vi "WAV_Binarize.vi"(10 "Data in":sgl[][](graph), 11 "format":T1) -> (2 "file string":string)   [LabVIEW 2022 SP3]
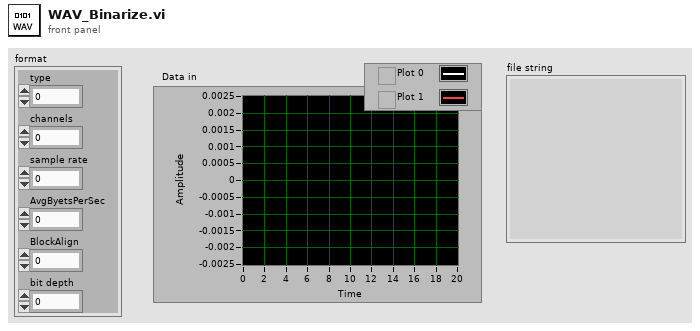
[diagram p1: front panel]
types:
  T1 = cluster{"type":u16, "channels":u16, "sample rate":u32, "AvgByetsPerSec":u32, "BlockAlign":u16, "bit depth":u16}
  T2 = enum16{"big-endian, network order", "native, host order", "little-endian"}
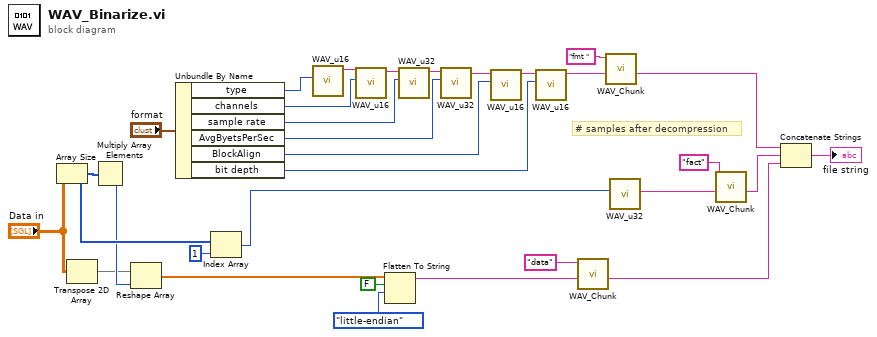
[diagram p0: block diagram]
diagram:
  # "# samples after decompression"
  n1 = Array Size(array="Data in") -> (size(s)=w17:i32[])
  n2 = Transpose 2D Array(2D array="Data in") -> (transposed array=w11:sgl[][])
  n3 = Multiply Array Elements(1:w17) -> (0:w13:i32)
  n4 = Reshape Array(w11, w13) -> (w20:sgl[])
  n5 = Unbundle By Name("format") -> ("type"=w23:u16, "channels"=w25:u16, "sample rate"=w30:u32, "AvgByetsPerSec"=w22:u32, "BlockAlign"=w29:u16, "bit depth"=w9:u16)
  n6 = Index Array(array=w17, index=1) -> (element=w31:i32)
  n7 = call "WAV_u16.vi"("u16"=w23) -> ("String out"=w24:string)  [unwired: 10 in]
  n8 = call "WAV_u16.vi"("u16"=w25, "String in"=w24) -> ("String out"=w26:string)  [unwired: 9 in]
  n9 = Flatten To String(anything=w20, prepend array or string size? (T)=FALSE, byte order (0:big-endian, network order)=T2."little-endian") -> (data string=w8:string)  [unwired: 1 in, 2 out]
  n10 = call "WAV_u32.vi"("u32"=w30, "String in"=w26) -> ("String out"=w21:string)  [unwired: 9 in]
  n11 = call "WAV_u32.vi"("u32"=w22, "String in"=w21) -> ("String out"=w28:string)  [unwired: 9 in]
  n12 = call "WAV_u16.vi"("u16"=w29, "String in"=w28) -> ("String out"=w27:string)  [unwired: 9 in]
  n13 = call "WAV_u16.vi"("u16"=w9, "String in"=w27) -> ("String out"=w4:string)  [unwired: 9 in]
  n14 = call "WAV_Chunk.vi"("data string"=w8, "string"="data") -> ("String out"=w7:string)  [unwired: 9 in]
  n15 = call "WAV_Chunk.vi"("data string"=w4, "string"="fmt ") -> ("String out"=w5:string)  [unwired: 9 in]
  n16 = call "WAV_u32.vi"("u32"=w31) -> ("String out"=w3:string)  [unwired: 10 in]
  n17 = call "WAV_Chunk.vi"("data string"=w3, "string"="fact" ("String")) -> ("String out"=w1:string)  [unwired: 9 in]
  n18 = Concatenate Strings(w5, w1, w7) -> (→"file string":string)
